vi "Query Library for Module Info.vi"(11 "error in (no error)":errorcluster) -> (15 "error out":errorcluster)   [LabVIEW 2020, in "DQMH_API.lvclass"]
uses:
  <resource>/Framework/Providers/Open_GDS/UML/DQMH_API_class/DQMH_API.lvclass
panel:
  in  "Library":refnum<vi>
  out "Module Locked?":bool
  out "Module Dirty?":bool
  out "Valid DQMH Module?":bool
  out "Module Info":T1
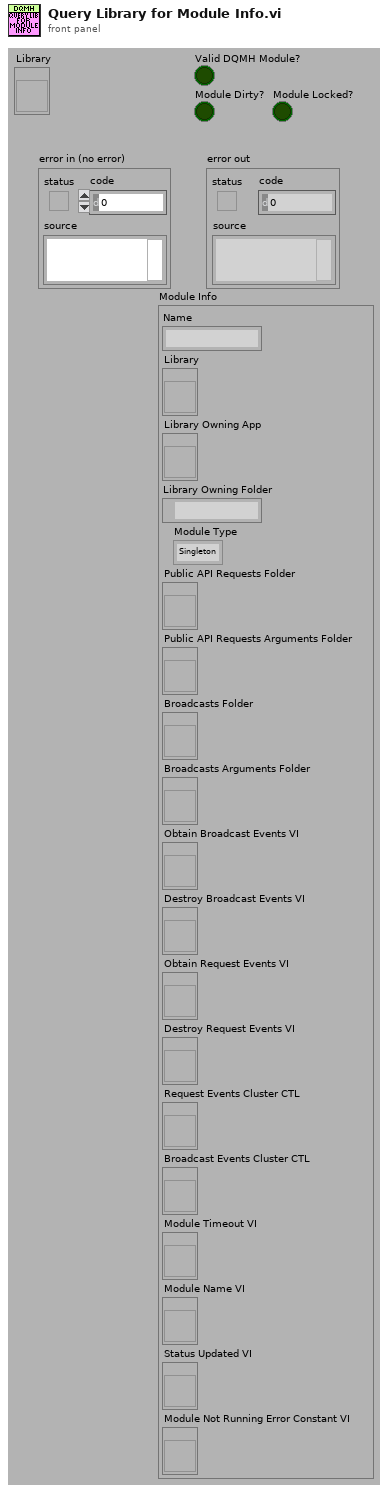
[diagram p1: front panel]
types:
  T1 = cluster{"Name":string, "Library":refnum<vi>, "Library Owning App":refnum<vi>, "Library Owning Folder":path, "Module Type":enum16{"Singleton", "Cloneable"}, "Public API Requests Folder":refnum<vi>, "Public API Requests Arguments Folder":refnum<vi>, "Broadcasts Folder":refnum<vi>, "Broadcasts Arguments Folder":refnum<vi>, "Obtain Broadcast Events VI":refnum<vi>, "Destroy Broadcast Events VI":refnum<vi>, "Obtain Request Events VI":refnum<vi>, "Destroy Request Events VI":refnum<vi>, "Request Events Cluster CTL":refnum<vi>, "Broadcast Events Cluster CTL":refnum<vi>, "Module Timeout VI":refnum<vi>, "Module Name VI":refnum<vi>, "Status Updated VI":refnum<vi>, "Module Not Running Error Constant VI":refnum<vi>}
  T2 = typedef "DQMH_API.lvclass/ObjectAttributes.ctl" = cluster{"Get Module Type Info":refnum<vi>, "Script New Module":refnum<vi>, "Script New Event":refnum<vi>, "Query Library for Module Info":refnum<vi>, "Parse Project for DQMH Modules":refnum<vi>, "Get All Events in Module":refnum<vi>}
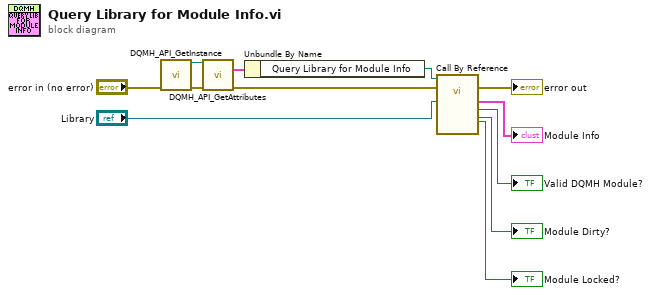
[diagram p0: block diagram]
diagram:
  n1 = call <resource>:"DQMH_API_GetInstance.vi"("error in (no error)"="error in (no error)") -> ("reference out"=w8:refnum<class "DQMH_API.lvclass">, "error out"=w7:errorcluster)  [unwired: 10 in, 3 out]
  n2 = call <resource>:"DQMH_API_GetAttributes.vi"("reference in"=w8, "error in (no error)"=w7) -> ("Data"=w9:T2, "error out"=w5:errorcluster)  [unwired: 10 in, 2 out]
  n3 = Unbundle By Name(w9) -> ("Query Library for Module Info"=w6:refnum<vi>)
  n4 = call-by-ref "?"(reference=w6, error in=w5, "Library"="Library") -> (error out=→"error out":errorcluster, "Module Dirty?"=→"Module Dirty?":bool, "Valid DQMH Module?"=→"Valid DQMH Module?":bool, "Module Info"=→"Module Info":T1, "Module Locked?"=→"Module Locked?":bool)  [unwired: 6 in, 2 out]
